vi "Get Process Interface Actions.vi"(8 "error in (no error)":errorcluster {"code" format="Error %.0f"}, 11 "VIDoc Printer In":refnum<class "VIDoc Printer.lvclass">) -> (0 "error out":errorcluster {"code" format="Error %.0f"}, 2 "Process Interface Actions":T1[](array[typedef]), 3 "VIDoc Printer Out":refnum<class "VIDoc Printer.lvclass">)   [LabVIEW 2023, in "VIDoc Printer.lvlib" / "VIDoc Printer.lvclass"]
uses:
  VIDoc Printer.lvclass
  VIDoc Printer.lvclass/VIDoc Printer.ctl
  Controls/Process Interfaces Enum.ctl
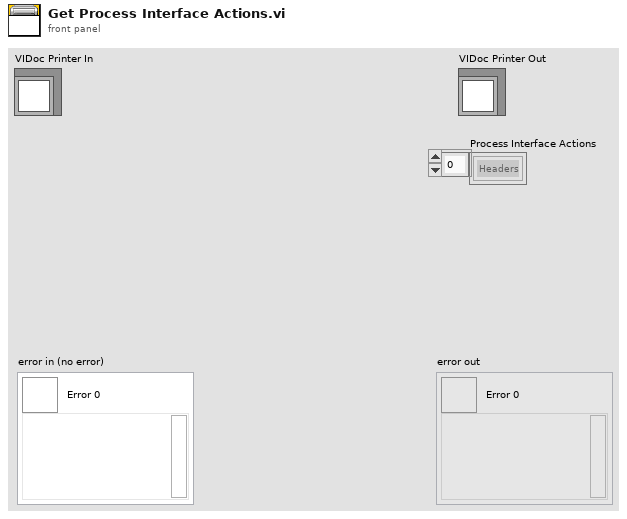
[diagram p1: front panel]
types:
  T1 = typedef "VIDoc Printer.lvlib/VIDoc Printer.lvclass/Process Interfaces Enum.ctl" = enum16{"Headers", "Memory", "By List", "Description", "Inheritance", "Inheritance Parent Interfaces", "Inheritance Friends", "Methods", "Controls"}
  T2 = typedef "VIDoc Printer.lvlib/Printer Settings.lvclass/Detail Level Enum.ctl" = enum16{"None", "Minimal", "Standard", "Full"}
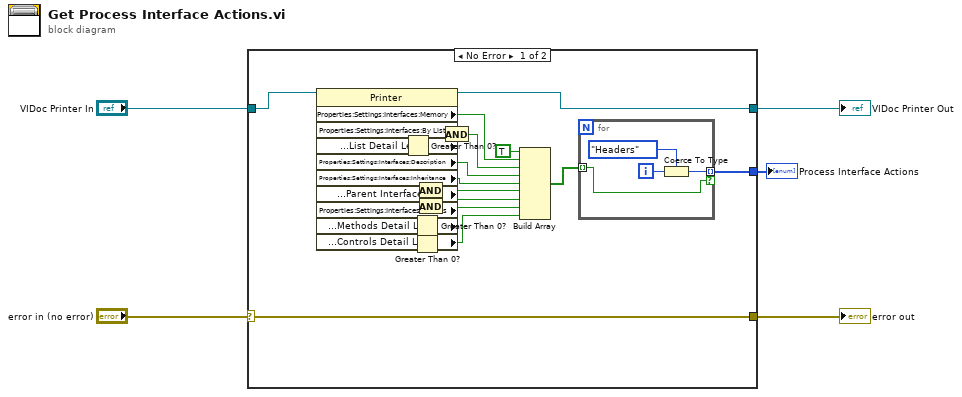
[diagram p0: block diagram]
diagram:
  n1 = case shown="No Error" "error in (no error)" {
    selector: "error in (no error)" -> [w26 w32]
    tunnel: [w26 w32] -> w4
    tunnel: [w23 w31] -> w2
    tunnel: "VIDoc Printer In" -> [w24 w31]
    tunnel: [w21 _] -> w1
    frame No Error {
      n2 = property class="Printer"(reference=w24) -> (reference out=w23:refnum<class "VIDoc Printer.lvclass">, "Properties:Settings:Interfaces:Memory"=w16:bool, "Properties:Settings:Interfaces:By List"=w25:bool, "Properties:Settings:Interfaces:List Detail Level"=w20:T2, "Properties:Settings:Interfaces:Description"=w15:bool, "Properties:Settings:Interfaces:Inheritance"=w12:bool, "Properties:Settings:Interfaces:Parent Interfaces"=w14:bool, "Properties:Settings:Interfaces:Friends"=w13:bool, "Properties:Settings:Interfaces:Methods Detail Level"=w9:T2, "Properties:Settings:Interfaces:Controls Detail Level"=w8:T2)  [unwired: 1 in, 1 out]
      n3 = Greater Than 0?(x=w20) -> (x > 0?=w18:bool)
      n4 = Greater Than 0?(x=w9) -> (x > 0?=w7:bool)
      n5 = Greater Than 0?(x=w8) -> (x > 0?=w6:bool)
      n6 = And(x=w12, y=w14) -> (x .and. y?=w11:bool)
      n7 = And(x=w12, y=w13) -> (x .and. y?=w10:bool)
      n8 = And(x=w25, y=w18) -> (x .and. y?=w19:bool)
      n9 = Build Array(TRUE ("element"), w16, w19, w15, w12, w11, w10, w7, w6) -> (w22:bool[])
      n10 = for {
        tunnel: w22 -> [w27] mode=indexing
        tunnel: [w28] -> w21 mode=indexing if=w27
        i -> [w29]
        n11 = Coerce To Type(0:w29, 1:Process_Interfaces_Enum."Headers") -> (2:w28:T1)
      }
    }
    frame Error {
    }
  }
  "error out" <- w4
  "VIDoc Printer Out" <- w2
  "Process Interface Actions" <- w1
